vi "Parse MS Packet.vi"(1 "Packet Measurement Data":string) -> (0 "Raw Height Data":i32[](array[numeric]))   [LabVIEW 2016]
doc: "Iterates URG-04LX MS (2-byte) packet data in search of height measurements."
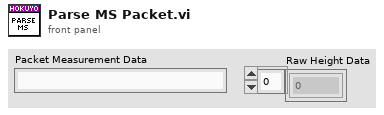
[diagram p1: front panel]
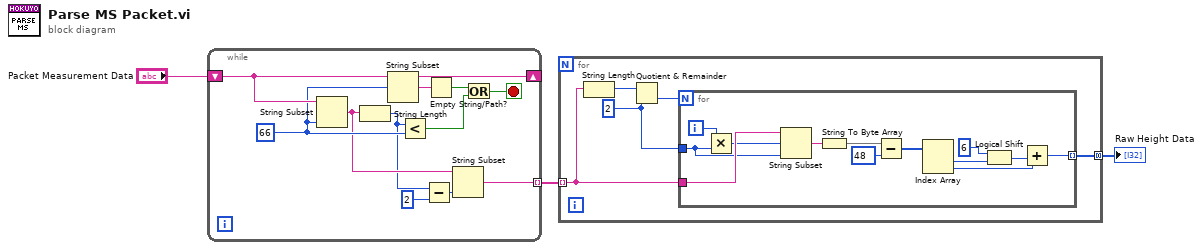
[diagram p0: block diagram]
diagram:
  n1 = while {
    shift-right: [w9] -> _
    shift-left: "Packet Measurement Data" -> [w14]
    tunnel: [w4] -> w2 mode=indexing
    stop <- w10 stop-if-true
    w13 = 66 ("length (rest)")
    n2 = String Subset(string=w14, length (rest)=w13) -> (substring=w8:string)  [unwired: 1 in]
    n3 = String Length(string=w8) -> (length=w6:i32)
    n4 = String Subset(string=w14, offset (0)=w13) -> (substring=w9:string)  [unwired: 1 in]
    n5 = Less?(x=w6, y=w13) -> (x < y?=w11:bool)
    n6 = Subtract(x=w6, y=2) -> (x-y=w7:i32)
    n7 = Empty String/Path?(string/path=w9) -> (empty?=w12:bool)
    n8 = String Subset(string=w8, length (rest)=w7) -> (substring=w4:string)  [unwired: 1 in]
    n9 = Or(x=w12, y=w11) -> (x .or. y?=w10:bool)
  }
  n10 = for {
    tunnel: w2 -> [w17] mode=indexing
    tunnel: [w15] -> w1 mode=concatenating
    w16 = 2 ("y")
    n11 = String Length(string=w17) -> (length=w19:i32)
    n12 = Quotient & Remainder(x=w19, y=w16) -> (floor(x/y)=w18:i32)  [unwired: 1 out]
    n13 = for {
      N: w18 -> [_]
      tunnel: w17 -> [w32]
      tunnel: w16 -> [w21]
      tunnel: [w22] -> w15 mode=indexing
      i -> [w20]
      n14 = Multiply(x=w20, y=w21) -> (x*y=w31:i32)
      n15 = String Subset(string=w32, offset (0)=w31, length (rest)=w21) -> (substring=w23:string)
      n16 = String To Byte Array(string=w23) -> (unsigned byte array=w30:u8[])
      n17 = Subtract(x=w30, y=48) -> (x-y=w25:i32[])
      n18 = Index Array(array=w25) -> (element #1=w26:i32, element #2=w29:i32)  [unwired: 2 in]
      n19 = Logical Shift(y=i8 6, x=w26) -> (x << y=w28:i32)
      n20 = Add(x=w28, y=w29) -> (x+y=w22:i32)
    }
  }
  "Raw Height Data" <- w1
